vi "Read Responder.vi"(8 "error in (no error)":errorcluster, 11 "BaseDriver in":refnum<class "BaseDriver.lvclass">) -> (0 "error out":errorcluster, 2 "Responder":refnum<class "BaseResponder.lvclass">, 3 "BaseDriver out":refnum<class "BaseDriver.lvclass">)   [LabVIEW 2013, in "BaseDriver.lvclass"]
doc: "When there is no data to read and no data to send to the remote destination, the driver will wait for either to be available, according to the Idle Read property. It will wait for Poll interval milliseconds before checking again."
uses:
  BaseDriver.lvclass
  Responder/BaseResponder/BaseResponder.lvclass
  BaseDriver.lvclass/BaseDriver.ctl
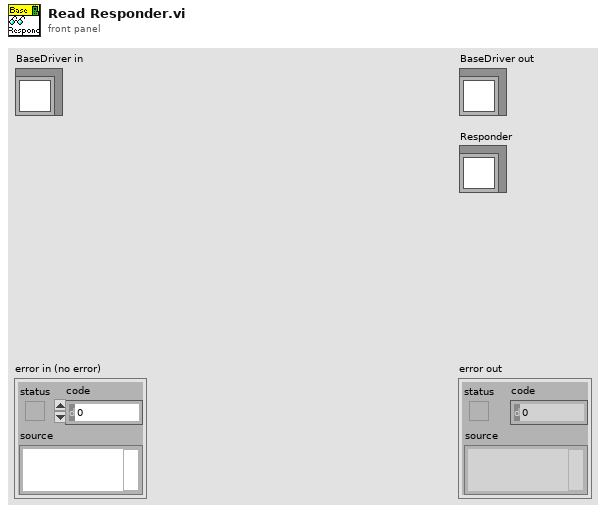
[diagram p1: front panel]
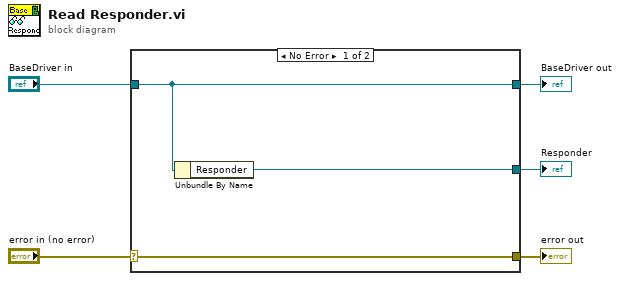
[diagram p0: block diagram]
diagram:
  n1 = case shown="No Error" "error in (no error)" {
    selector: "error in (no error)" -> [w8 w9]
    tunnel: [w8 w9] -> w4
    tunnel: [w7 w10] -> w2
    tunnel: "BaseDriver in" -> [w7 w10]
    tunnel: [w6 _] -> w1
    frame No Error {
      n2 = Unbundle By Name(w7) -> ("Responder"=w6:refnum<class "BaseResponder.lvclass">)
    }
    frame Error {
    }
  }
  "error out" <- w4
  "BaseDriver out" <- w2
  "Responder" <- w1
